vi "Configure Multi Eval Meas Frequency Accuracy Limit.vi"(5 "Freq Accuracy kHz (On)":bool=TRUE, 6 "Freq Accuracy ppm (On)":bool=TRUE, 7 "Freg Accuracy kHz (0)":dbl format="%^.3e", 8 "error in (no error)":errorcluster, 9 "Freg Accuracy ppm (0)":dbl format="%^.3e", 10 "Instance (1)":i32=1, 11 "VISA resource name":refnum<visa-resource-name>) -> (0 "error out":errorcluster, 3 "VISA resource name out":refnum<visa-resource-name>)   [LabVIEW 2020, in "Rohde&Schwarz CMP LR WPAN Measurement.lvlib"]
doc: "Defines the upper limit for the frequency accuracy.\n\nOrder of paramaters:\n<FreqAccuracyppm>\n<FreqAccuracykHz>\n<FreqAccppmEnble>\n<FreqAcckHzEnble>\n\nAttribute:\n-\n\nRemote-control command:\nCONFigure:WPAN:MEAS<i>:MEValuation:LIMit:FACCuracy"
uses:
  <instrlib>/Rohde&Schwarz CMP LR WPAN Measurement/Rohde&Schwarz CMP LR WPAN Measurement.lvlib
  <instrlib>/Rohde&Schwarz CMP LR WPAN Measurement/Private/rsidr_core.llb/rsidr_core.lvlib
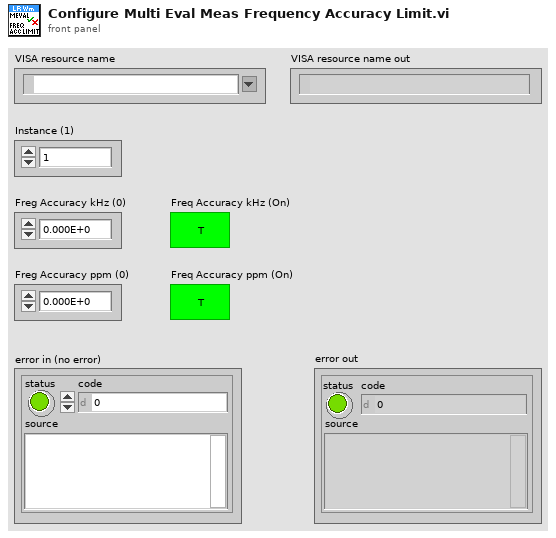
[diagram p1: front panel]
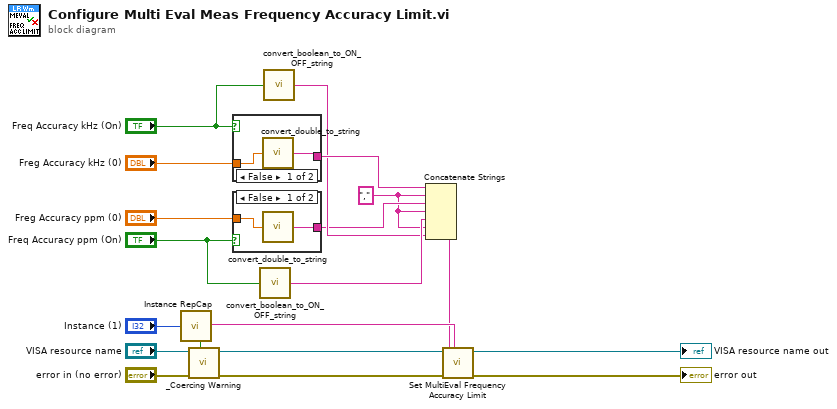
[diagram p0: block diagram]
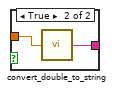
[diagram p2: hidden frame]
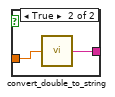
[diagram p3: hidden frame]
diagram:
  w1 = ","
  n1 = call <instrlib>:"Instance RepCap.vi"("Instance In"="Instance (1)") -> ("In Range?"=w19:bool, "RepCap Identifier Out"=w18:string)  [unwired: 1 in]
  n2 = call <instrlib>:"_Coercing Warning.vi"("In Range?"=w19, "error in (no error)"="error in (no error)", "VISA resource name"="VISA resource name") -> ("error out"=w11:errorcluster, "VISA resource name out"=w10:refnum<visa-resource-name>)  [unwired: 7 in]
  n3 = case shown="False" "Freq Accuracy kHz (On)" {
    tunnel: "Freg Accuracy kHz (0)" -> [w20 w22]
    tunnel: [w21 w23] -> w15
    frame False {
      n4 = call <instrlib>:"convert_double_to_string.vi"("double in"=w20) -> ("string out"=w21:string)  [unwired: 4 in]
    }
    frame True {
      n5 = call <instrlib>:"convert_double_to_string.vi"("double in"=w22) -> ("string out"=w23:string)  [unwired: 4 in]
    }
  }
  n6 = case shown="False" "Freq Accuracy ppm (On)" {
    tunnel: "Freg Accuracy ppm (0)" -> [w24 w27]
    tunnel: [w25 w26] -> w2
    frame False {
      n7 = call <instrlib>:"convert_double_to_string.vi"("double in"=w24) -> ("string out"=w25:string)  [unwired: 4 in]
    }
    frame True {
      n8 = call <instrlib>:"convert_double_to_string.vi"("double in"=w27) -> ("string out"=w26:string)  [unwired: 4 in]
    }
  }
  n9 = call <instrlib>:"convert_boolean_to_ON_OFF_string.vi"("boolean value in"="Freq Accuracy ppm (On)") -> ("string value out"=w5:string)  [unwired: 4 in]
  n10 = call <instrlib>:"convert_boolean_to_ON_OFF_string.vi"("boolean value in"="Freq Accuracy kHz (On)") -> ("string value out"=w4:string)  [unwired: 4 in]
  n11 = Concatenate Strings(w15, w1, w2, w1, w5, w1, w4) -> (w14:string)
  n12 = call "Set MultiEval Frequency Accuracy Limit"("Repeated Capabilities"=w18, "error in (no error)"=w11, "MultiEval Frequency Accuracy Limit ()"=w14, "instrument handle"=w10) -> ("error out"=→"error out":errorcluster, "instrument handle out"=→"VISA resource name out":refnum<visa-resource-name>)  [unwired: 6 in]
